vi "read_NI - stability.vi"(6 "error in":errorcluster) -> (0 "all_pds":dbl[](array[numeric]), 1 "-pd3/pd1":dbl, 2 "pd3/pd1":dbl, 3 "fpga-ref-out":refnum<k20>, 4 "error out":errorcluster)   [LabVIEW 2024]
uses:
  <vilib>/FPGAPlugInAG/NI 9147/niLvFpga_Open_NI 9147.vi
  <vilib>/rvi/interface/common/dynamic/niFpgaDynamicAddResources.vi
  <vilib>/Utility/error.llb/Error Cluster From Error Code.vi
  <vilib>/rvi/errors/niLvFpgaAdjustHostInterfaceError.vi
  <vilib>/FPGAPlugInAG/Dynamic/niLvFpga_Run_Dynamic.vi
  <vilib>/FPGAPlugInAG/Dynamic/niLvFpga_Close_Dynamic.vi
  <vilib>/rvi/interface/nirviOpenFPGA/nirviOpenFPGA.xnode
  FPGA Bitfiles/dircdaq-automate_FPGATarget_fpga_RyAY8MzD2n8.lvbitx
  fpga.vi
  <vilib>/rvi/interface/nirviReadWriteControl/nirviReadWriteControl.xnode
  <vilib>/rvi/interface/nirviMethod/nirviMethod.xnode
  <vilib>/rvi/interface/nirviCloseFPGA/nirviCloseFPGA.xnode
  <vilib>/Analysis/NI_AALBase.lvlib
  NiFpgaLv.dll
  <vilib>/rvi/interface/Simulation/niFpgaSimulationCallBeginRW.vi
panel:
  out "out":string
  out "log-error":errorcluster
  out "spreadsheet string":string
  out "appended array":string[](array[string])
  out "Current Time:":string
  in  "stop":bool
  out "pd2/pd1":dbl
  out "ch2-sd":dbl format="%^#_6g"
  out "ch2-avg":dbl format="%^#_6g"
  out "ch1-sd":dbl format="%^#_6g"
  out "ch1-avg":dbl format="%^#_6g"
  out "ch0-sd":dbl format="%^#_6g"
  out "ch0-avg":dbl format="%^#_6g"
  out "fpga-heartbeat":bool
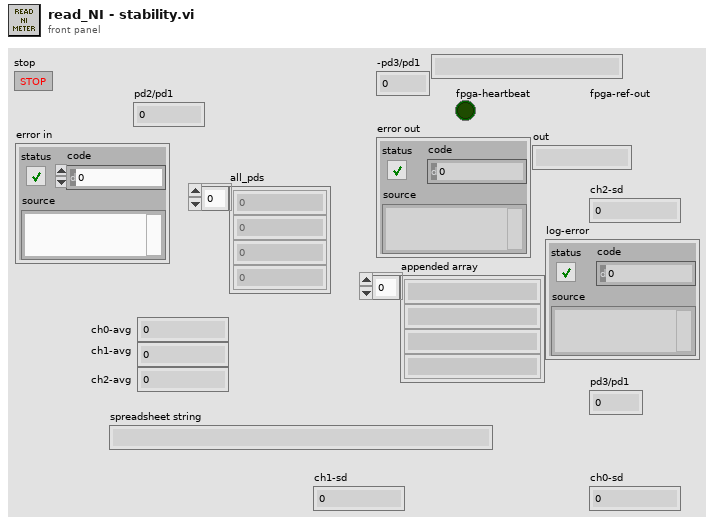
[diagram p1: front panel]
types:
  T1 = enum8{"High Speed", "Best 60 Hz Rejection", "Best 50 Hz Rejection", "High Resolution"}
  T2 = enum16{"open", "replace", "create", "open or create", "replace or create", "replace or create with confirmation"}
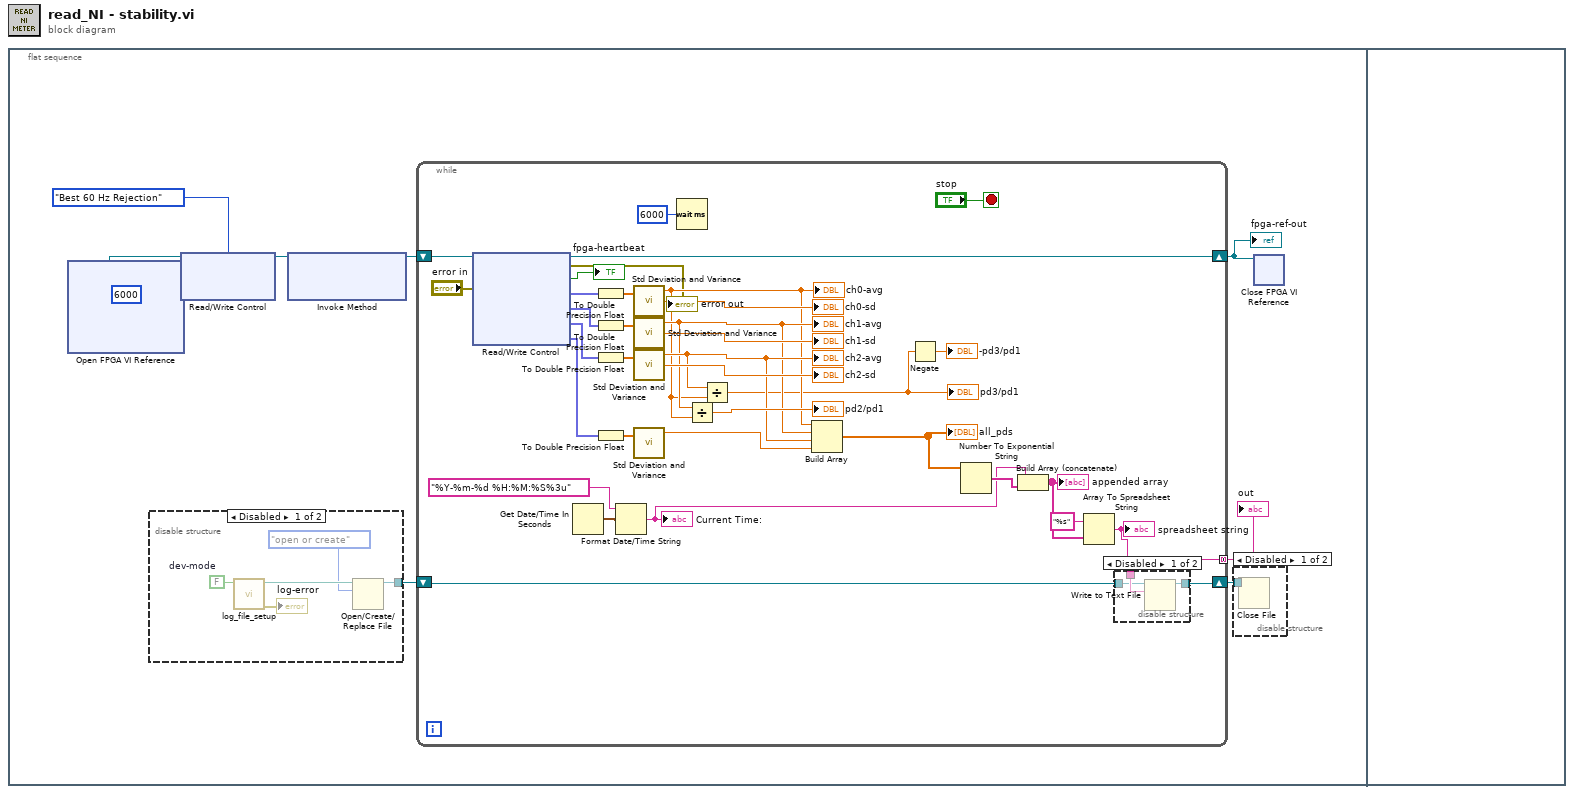
[diagram p0: block diagram]
diagram:
  n1 = flat-sequence {
    frame #0 {
      n2 = xnode "Open FPGA VI Reference"() -> ("FPGA VI Reference Out"=w7:refnum<k20>)  [unwired: 2 in, 1 out]
      n3 = disable-structure shown="Disabled" {
        disable-tunnel: [w12 _] -> w6
        frame Disabled {
          w14 = FALSE  # dev-mode
          n4 = call "log_file_setup.vi"("dev-mode"=w14) -> ("error out"=→"log-error":errorcluster, "appended path"=w13:path)  [unwired: 8 in, 1 out]
          n5 = Open/Create/Replace File(file path (use dialog)=w13, operation (0:open)=T2."open or create") -> (refnum out=w12:refnum<file>)  [unwired: 4 in, 2 out]
        }
        frame Enabled {
        }
      }
      n6 = xnode "Read/Write Control"("FPGA VI Reference In"=w7, "NI-mode"=T1."Best 60 Hz Rejection", "daq-period-us"=u32 6000) -> ("FPGA VI Reference Out"=w3:refnum<k20>)  [unwired: 1 in, 1 out]
      n7 = xnode "Invoke Method"("FPGA VI Reference In"=w3) -> ("FPGA VI Reference Out"=w9:refnum<k20>)  [unwired: 2 in, 1 out]
      n8 = while {
        shift-right: [w31] -> w8
        shift-left: w9 -> [w32]
        tunnel: [w20] -> w4 mode=concatenating
        shift-right: [w21] -> w5
        shift-left: w6 -> [w19]
        stop <- "stop" stop-if-true
        n9 = xnode "Read/Write Control"("FPGA VI Reference In"=w32, "error in"="error in") -> ("FPGA VI Reference Out"=w31:refnum<k20>, "error out"=→"error out":errorcluster, "fpga-heartbeat"=→"fpga-heartbeat":bool, "ch0"=w37:fxp<+/-,32,-1>[], "ch1"=w40:fxp<+/-,32,-1>[], "ch2"=w42:fxp<+/-,32,-1>[], "ch3"=w17:fxp<+,32,14>[])
        n10 = Get Date/Time In Seconds() -> (seconds since 1Jan1904=w28:timestamp)
        n11 = To Double Precision Float(number=w37) -> (double precision float=w39:dbl[])
        n12 = To Double Precision Float(number=w40) -> (double precision float=w38:dbl[])
        n13 = To Double Precision Float(number=w42) -> (double precision float=w41:dbl[])
        n14 = To Double Precision Float(number=w17) -> (double precision float=w18:dbl[])
        n15 = Format Date/Time String(time format string (%c)="%Y-%m-%d %H:%M:%S%3u", seconds (now)=w28) -> (date/time string=w24:string)  [unwired: 1 in]
        "Current Time:" <- w24
        n16 = call <vilib>:"Std Deviation and Variance.vi"("X"=w39) -> ("mean"=w44:dbl, "standard deviation"=→"ch0-sd":dbl)  [unwired: 1 in, 1 out]
        "ch0-avg" <- w44
        n17 = call <vilib>:"Std Deviation and Variance.vi"("X"=w38) -> ("mean"=w46:dbl, "standard deviation"=→"ch1-sd":dbl)  [unwired: 1 in, 1 out]
        "ch1-avg" <- w46
        n18 = call <vilib>:"Std Deviation and Variance.vi"("X"=w41) -> ("mean"=w47:dbl, "standard deviation"=→"ch2-sd":dbl)  [unwired: 1 in, 1 out]
        "ch2-avg" <- w47
        n19 = call <vilib>:"Std Deviation and Variance.vi"("X"=w18) -> ("mean"=w16:dbl)  [unwired: 1 in, 2 out]
        n20 = Wait (ms)(milliseconds to wait=u32 6000) -> ()  [unwired: 1 out]
        n21 = Divide(x=w46, y=w44) -> (x/y=→"pd2/pd1":dbl)
        n22 = Divide(x=w47, y=w44) -> (x/y=w35:dbl)
        "pd3/pd1" <- w35
        n23 = Build Array(w44, w46, w47, w16) -> (w26:dbl[])
        "all_pds" <- w26
        n24 = Negate(x=w35) -> (-x=→"-pd3/pd1":dbl)
        n25 = Number To Exponential String(number=w26) -> (E-format string=w25:string[])  [unwired: 3 in]
        n26 = Build Array (concatenate)(w24, w25) -> (w23:string[])
        "appended array" <- w23
        n27 = Array To Spreadsheet String(array=w23, 3:"%s" ("format string")) -> (spreadsheet string=w20:string)  [unwired: 1 in]
        "spreadsheet string" <- w20
        n28 = disable-structure shown="Disabled" {
          disable-tunnel: [w53 _] -> w21
          disable-tunnel: w20 -> [w52 _]
          disable-tunnel: w19 -> [w51 _]
          frame Disabled {
            n29 = Write to Text File(file (use dialog)=w51, text=w52) -> (refnum out=w53:refnum<file>)  [unwired: 2 in, 2 out]
          }
          frame Enabled {
          }
        }
      }
      "fpga-ref-out" <- w8
      "out" <- w4
      n30 = disable-structure shown="Disabled" {
        disable-tunnel: w5 -> [w10 _]
        frame Disabled {
          n31 = Close File(refnum=w10) -> ()  [unwired: 1 in, 2 out]
        }
        frame Enabled {
        }
      }
      n32 = xnode "Close FPGA VI Reference"("FPGA VI Reference In"=w8) -> ()  [unwired: 1 in, 1 out]
    }
    frame #1 {
    }
  }
